vi "User_Metadata.vi"() -> ()   [LabVIEW 2020]
uses:
  ADAM Controls/Channel_names.ctl
  ADAM Controls/Calib_type_ADAM.ctl
  Anemometry/Anemometry Sub Vis/Controls/Preference_Mode.ctl
  ADAM Controls/Channel_State.ctl
  ADAM Controls/Module_type_ADAM.ctl
  ADAM Controls/Update_scan_value.ctl
  Anemometry/Anemometry Sub Vis/Globals/Preference_global.vi
  Anemometry/Anemometry Sub Vis/Globals/Constants_global.vi
  Anemometry/Anemometry Sub Vis/Globals/Meas_global.vi
  Anemometry/Anemometry Sub Vis/Globals/Trav_pos_global.vi
panel:
  out "Channel Name 13":string
  out "Channel Name 12":string
  out "Channel Name 11":string
  in  "Value 13":string
  in  "Value 12":string
  in  "Value 11":string
  in  "Menu 13":u16(ring) items=["Edit Strings", "20mm Cubes"]
  in  "Menu 12":u16(ring) items=["Edit Strings", "20mm Cubes"]
  in  "Menu 11":u16(ring) items=["Edit Strings", "20mm Cubes"]
  out "Rig Name":string="EnFlo Tunnel"
  in  "Edit Email Addresses":bool
  out "Email Addresses":string[](array[string])
  in  "Value 10":string
  in  "Value 9":string
  in  "Value 8":string
  in  "Value 7":string
  in  "Value 6":string
  in  "Menu 10":u16(ring) items=["Edit Strings", "20mm Cubes"]
  out "Channel Name 10":string
  in  "Menu 9":u16(ring) items=["Edit Strings", "None", "Ramp 29 x 390mm", "Ramp 9 x 175mm", "Rounded nose 18.2 x 55mm", "Rounded nose 9 x 150mm"]
  out "Channel Name 9":string
  in  "Menu 8":u16(ring) items=["Edit Strings", "20mm Cubes"]
  out "Channel Name 8":string
  in  "Menu 7":u16(ring) items=["Edit Strings", "0", "115", "65"]
  out "Channel Name 7":string
  in  "Menu 6":u16(ring) items=["Edit Strings", "0", "1", "16"]
  out "Channel Name 6":string
  out "Clear remaining channels":bool
  in  "Value 5":string
  in  "Menu 5":u16(ring) items=["Edit Strings", "0", "25", "6.25"]
  out "Channel Name 5":string
  in  "Value 4":string
  in  "Menu 4":u16(ring) items=["Edit Strings", "20 x 20mm", "40 x 40mm", "80 x 80mm", "None"]
  out "Channel Name 4":string
  in  "Value 3":string
  in  "Menu 3":u16(ring) items=["Edit Strings", "0", "10", "20", "Normal distribution with average = 10mm"]
  out "Channel Name 3":string
  in  "Value 2":string
  in  "Menu 2":u16(ring) items=["Edit Strings", "None", "Random blocks", "Uniform cube"]
  out "Channel Name 2":string
  in  "Modify User Channels":bool
  out "Channel No":i32
  out "First Loop":bool
  out "Index":i32
  in  "Value 1":string
  in  "Menu 1":u16(ring) items=["Edit Strings", "Aligned", "None", "Staggered"]
  out "Channel Name 1":string
  in  "stop":bool
  in  "OK":bool
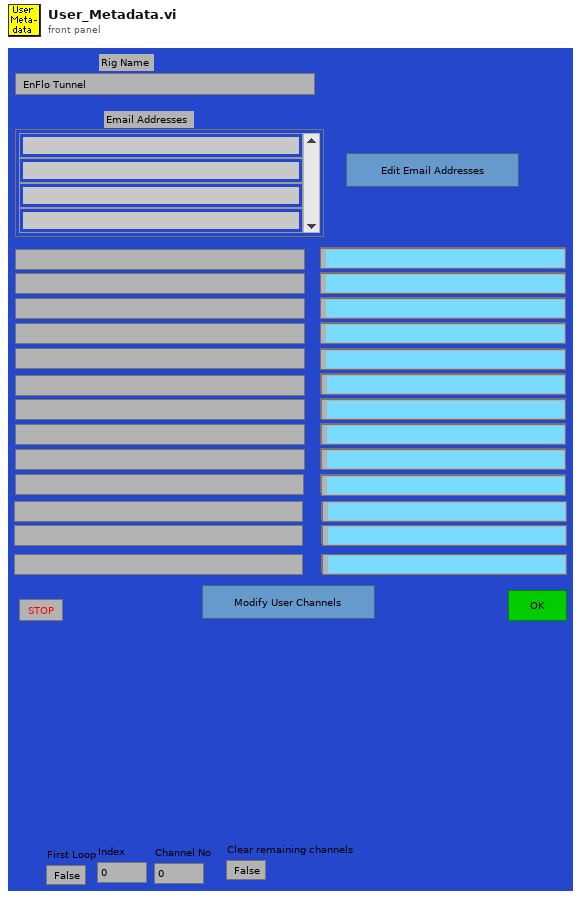
[diagram p1: front panel]
types:
  T1 = typedef "Channel_names.ctl" = enum16{"Active Only", "Active + Off", "All Channels"}
  T2 = typedef "Calib_type_ADAM.ctl" = string
  T3 = typedef "Preference_Mode.ctl" = enum16{"Load Preferences from file", "Save Preferences to file", "Load, Edit then Save"}
  T4 = typedef "Channel_State.ctl" = enum16{"On", "Off", "Always On", "Always Off"}
  T5 = typedef "Module_type_ADAM.ctl" = string
  T6 = typedef "Ch_description_ADAM.ctl" = cluster{"Ch Name":string, "Type":T5, "Function":T7, "Ch State":T4, "Calibration type":T2, "A":dbl, "B":dbl, "C":dbl, "D":dbl, "Comments":string, "Address":T8, "String":string, "Duty":u16}
  T7 = typedef "Function_ADAM.ctl" = enum16{"Analogue Input", "Digital Input", "Event counter", "Event rate", "Analogue Output", "Digital Output", "Relay Output"}
  T8 = typedef "Address.ctl" = cluster{"Main":i32, "Ch.":i32, "Sub":i32, "Port Name":string}
  T9 = typedef "Update_scan_value.ctl" = cluster{"Channel Name":string, "New Value":dbl}
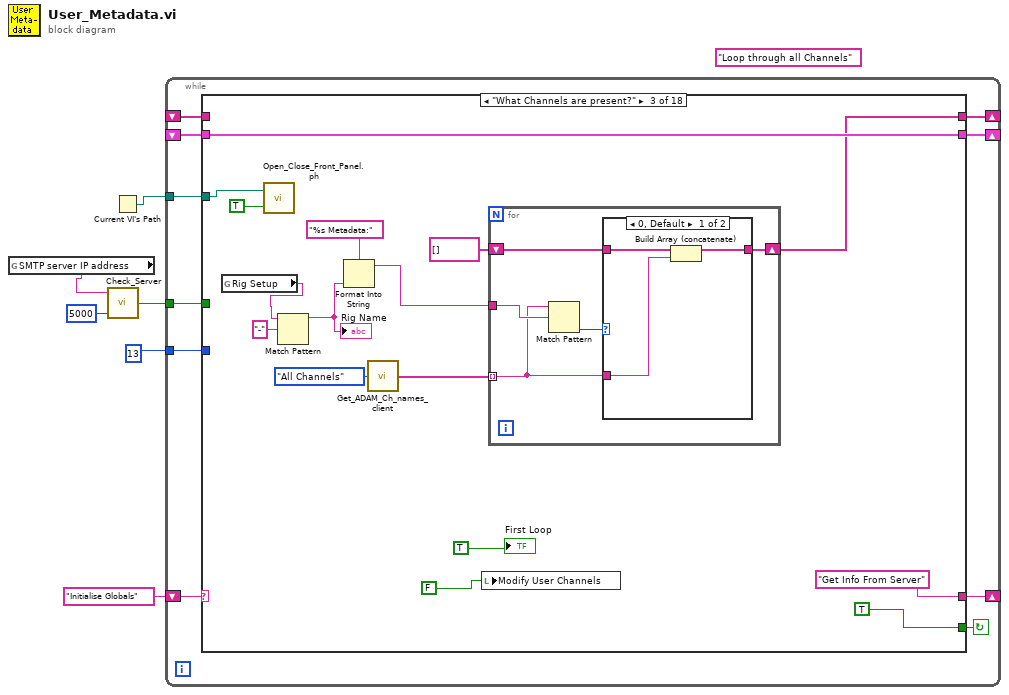
[diagram p0: block diagram]
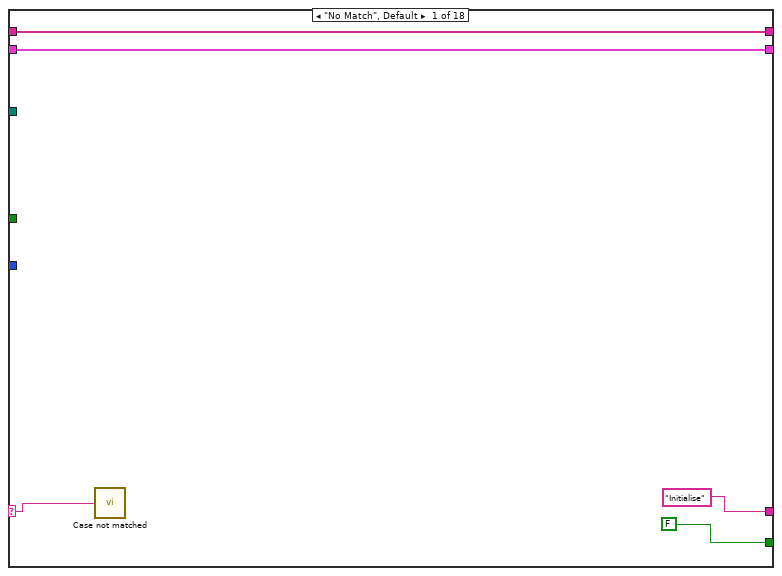
[diagram p2: hidden frame]
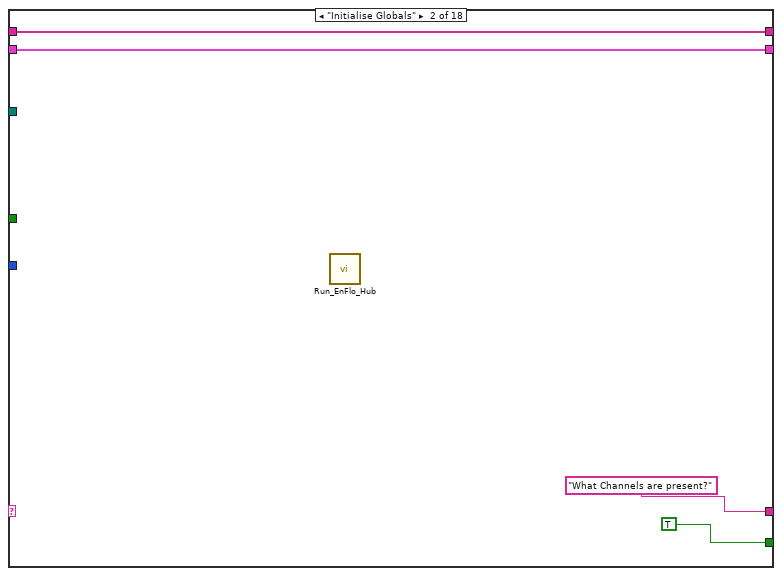
[diagram p3: hidden frame]
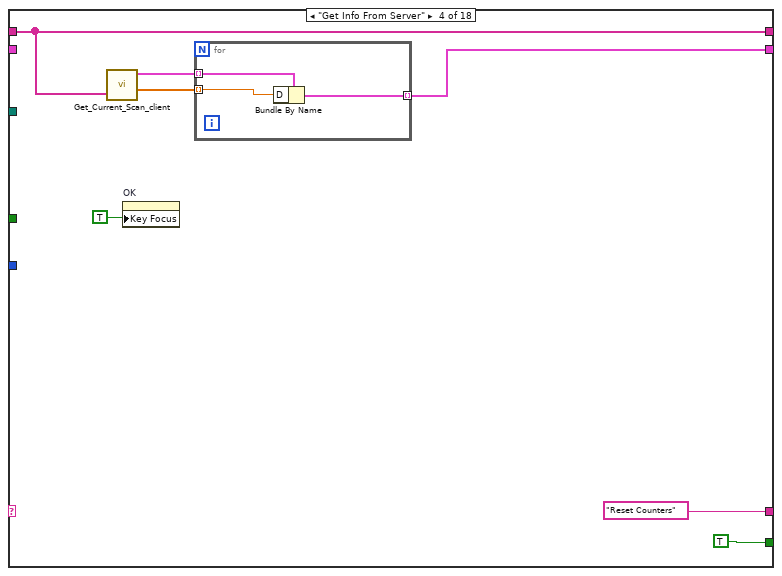
[diagram p5: hidden frame]
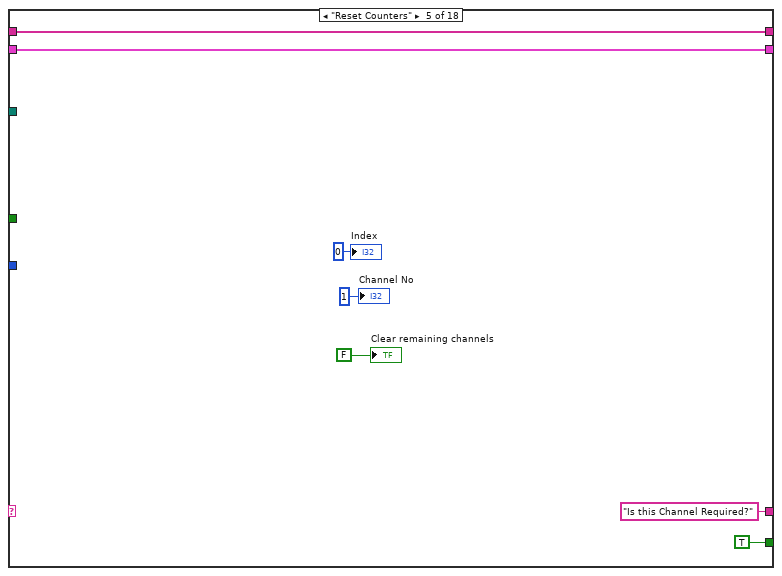
[diagram p6: hidden frame]
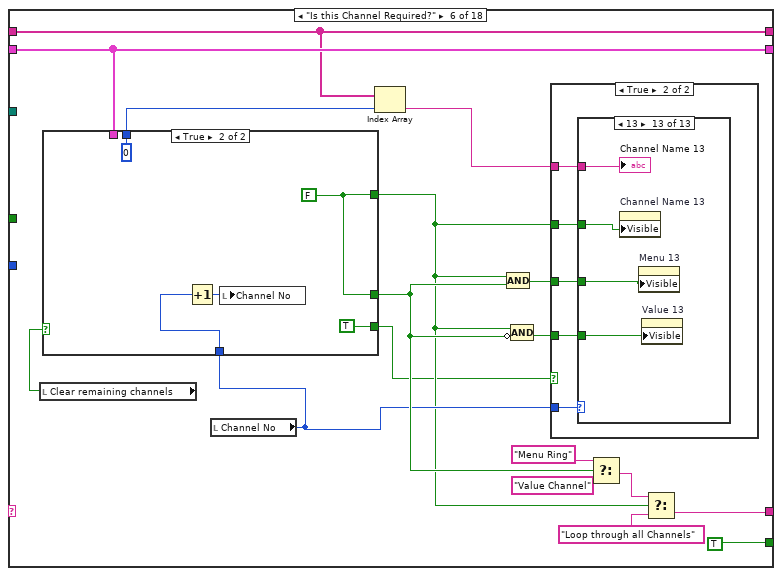
[diagram p7: hidden frame]
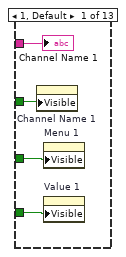
[diagram p9: hidden frame]
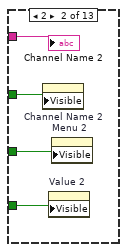
[diagram p10: hidden frame]
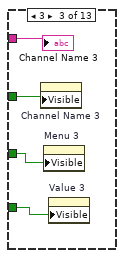
[diagram p11: hidden frame]
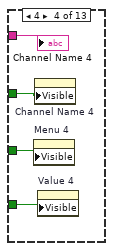
[diagram p12: hidden frame]
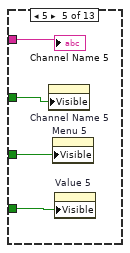
[diagram p13: hidden frame]
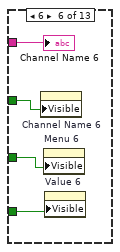
[diagram p14: hidden frame]
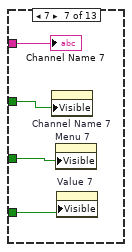
[diagram p15: hidden frame]
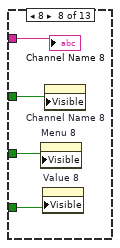
[diagram p16: hidden frame]
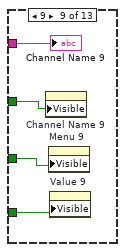
[diagram p17: hidden frame]
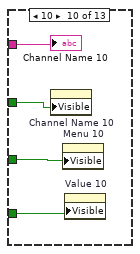
[diagram p18: hidden frame]
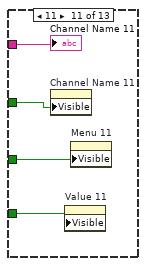
[diagram p19: hidden frame]
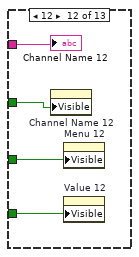
[diagram p20: hidden frame]
diagram:
  (unwired) "Loop through all Channels"
  n1 = global read "Preference_global.vi" "SMTP server IP address"() -> (w2:string)
  n2 = call "Check_Server.vi"("timeout ms (60000)"=5000, "address"=w2) -> ("OK"=w1:bool)  [unwired: 3 out]
  n3 = Current VI's Path() -> (path=w4:path)
  n4 = while {
    tunnel: 13 -> [w9]
    shift-left: _ -> [w12]
    shift-right: [w11] -> _
    shift-left: _ -> [w13]
    shift-right: [w14] -> _
    shift-left: "Initialise Globals" -> [w15]
    shift-right: [w10] -> _
    tunnel: w4 -> [w8]
    tunnel: w1 -> [w7]
    stop <- w16 continue-if-true
    n5 = case shown="\"What Channels are present?\"" w15 {
      selector: w15 -> [w17 _ _ _ _ _ _ _ _ _ _ _ _ _ _ _ _ _]
      tunnel: [FALSE TRUE TRUE TRUE TRUE ("T button?") TRUE TRUE TRUE TRUE TRUE TRUE TRUE TRUE TRUE ("T button?") TRUE ("T button?") TRUE ("T button?") TRUE ("T button?") FALSE ("T button?")] -> w16
      tunnel: ["Initialise" "What Channels are present?" "Get Info From Server" "Reset Counters" "Is this Channel Required?" w79 w173 "Increment Channel No" "Increment Channel No" "Loop through all Channels" w393 "What Channels are present?" "Reset Counters" w440 "Insert Values" "Update Server" w472 "End"] -> w10
      tunnel: [w19 w23 w39 w52 w64 w83 w165 w300 w321 w391 w404 w425 w430 w450 w457 w460 w473 w517] -> w14
      tunnel: w13 -> [w19 w23 w39 _ w64 w83 w166 w299 w322 w391 w404 w425 w431 w450 w457 w458 w473 w517]
      tunnel: w12 -> [w18 w22 _ w55 w65 w73 w185 w304 w332 w390 w409 w426 _ w443 w455 w459 w474 w518]
      tunnel: [w18 w22 w35 w55 w65 w73 w185 w304 w332 w390 w409 w426 w429 w443 w455 w459 w474 w518] -> w11
      tunnel: w9 -> [_ _ _ _ _ _ _ _ _ _ w399 _ _ _ _ _ _ _]
      tunnel: w8 -> [_ _ w30 _ _ _ _ _ _ _ _ _ _ _ _ _ _ w515]
      tunnel: w7 -> [_ _ _ _ _ _ _ _ _ _ _ _ _ _ _ _ _ _]
      frame "No Match", Default {
        n6 = call "Case not matched.vi"("Case Name not Matched"=w17) -> ()
      }
      frame "Initialise Globals" {
        n7 = call "Run_EnFlo_Hub.vi"() -> ()  [unwired: 1 in, 7 out]
      }
      frame "What Channels are present?" {
        n8 = global read "Preference_global.vi" "Rig Setup"() -> (w27:string)
        n9 = call "Open_Close_Front_Panel.ph.vi"("Front Panel Window:Open"=TRUE, "VI path"=w30) -> ()  [unwired: 2 out]
        n10 = Match Pattern(string=w27, regular expression="-") -> (before substring=w26:string)  [unwired: 4 out]
        "Rig Name" <- w26
        n11 = Format Into String(format string="%s Metadata:" ("Format String"), w26) -> (resulting string=w32:string)  [unwired: 2 in, 1 out]
        n12 = call "Get_ADAM_Ch_names_client.vi"("Channel names set"=Channel_names."All Channels") -> ("Ch names"=w37:string[])
        n13 = local write "Modify User Channels"(FALSE ("Add a New Channel")) -> ()
        n14 = for {
          tunnel: w32 -> [w46]
          tunnel: w37 -> [w44] mode=indexing
          shift-right: [w42] -> w35
          shift-left: string[] [] -> [w43]
          n15 = Match Pattern(string=w44, regular expression=w46) -> (offset past match=w45:i32)  [unwired: 4 out]
          n16 = case shown="0, Default" w45 {
            tunnel: w44 -> [w49 _]
            tunnel: w43 -> [w48 w50]
            tunnel: [w47 w50] -> w42
            frame 0, Default {
              n17 = Build Array (concatenate)(w48, w49) -> (w47:string[])
            }
            frame -1 {
            }
          }
        }
        "First Loop" <- TRUE ("First Loop")
      }
      frame "Get Info From Server" {
        n18 = call "Get_Current_Scan_client.vi"("multipleChannels"=w55) -> ("Ch Description Array"=w54:T6[], "Numerical Values"=w53:dbl[])  [unwired: 2 in, 1 out]
        n19 = property on="OK" class="Bool"("Key Focus"=TRUE) -> ()  [unwired: 2 in, 2 out]
        n20 = for {
          tunnel: w54 -> [w60] mode=indexing
          tunnel: w53 -> [w59] mode=indexing
          tunnel: [w58] -> w52 mode=indexing
          n21 = Bundle By Name(cluster=w60, "D"=w59) -> (w58:T6)
        }
      }
      frame "Reset Counters" {
        "Index" <- 0 ("Index")
        "Channel No" <- 1 ("Channel No")
        "Clear remaining channels" <- FALSE ("Clear remaining channels")
      }
      frame "Is this Channel Required?" {
        n22 = local read "Clear remaining channels"() -> (w71:bool)
        n23 = local read "Channel No"() -> (w70:i32)
        n24 = case shown="True" w71 {
          tunnel: w83 -> [w156 _]
          tunnel: [w142 w161] -> w69
          tunnel: [w152 w161] -> w78
          tunnel: [w151 0 ("Index")] -> w74
          tunnel: w70 -> [_ w158]
          tunnel: [w149 TRUE] -> w68
          frame False {
            n25 = local read "Index"() -> (w151:i32)
            n26 = Index Array(array=w156, index=w151) -> (element=w155:T6)
            n27 = Unbundle By Name(w155) -> ("Address.Port Name"=w146:string, "A"=w148:dbl, "Calibration type"=w153:T2)
            n28 = Equal?(x=w153, y=T2 "Text" ("Calibration Type")) -> (x = y?=w152:bool)
            n29 = Not Equal?(x="DELETE", y=w146) -> (x != y?=w143:bool)
            n30 = Equal?(x=w148, y=1.0 ("x")) -> (x = y?=w144:bool)
            n31 = And(x=w143, y=w144) -> (x .and. y?=w142:bool)
            n32 = Compound Arithmetic op=AND(w142, TRUE ("Input")) -> (w149:bool)
          }
          frame True {
            w161 = FALSE
            n33 = Increment(x=w158) -> (x+1=w159:i32)
            n34 = local write "Channel No"(w159) -> ()
          }
        }
        n35 = Index Array(array=w73, index=w74) -> (element=w72:string)
        n36 = Compound Arithmetic op=AND(w69, w78) -> (w81:bool)
        n37 = Compound Arithmetic op=AND(w69, invert w78) -> (w82:bool)
        n38 = case shown="True" w68 {
          tunnel: w82 -> [_ w89]
          tunnel: w81 -> [_ w88]
          tunnel: w69 -> [_ w87]
          tunnel: w72 -> [_ w86]
          tunnel: w70 -> [_ w85]
          frame False {
          }
          frame True {
            n39 = case shown="13" w85 {
              tunnel: w87 -> [w91 w95 w99 w103 w107 w112 w116 w120 w124 w128 w133 w137 w141]
              tunnel: w89 -> [w93 w97 w101 w105 w109 w110 w114 w118 w122 w126 w130 w134 w138]
              tunnel: w88 -> [w92 w96 w100 w104 w108 w111 w115 w119 w123 w129 w131 w135 w139]
              tunnel: w86 -> [w90 w94 w98 w102 w106 w113 w117 w121 w125 w127 w132 w136 w140]
              frame 1, Default {
                n40 = property on="Channel Name 1" class="Str"("Visible"=w91) -> ()  [unwired: 2 in, 2 out]
                n41 = property on="Menu 1" class="Ring (strict)"("Visible"=w92) -> ()  [unwired: 2 in, 2 out]
                n42 = property on="Value 1" class="Str"("Visible"=w93) -> ()  [unwired: 2 in, 2 out]
                "Channel Name 1" <- w90
              }
              frame 2 {
                n43 = property on="Channel Name 2" class="Str"("Visible"=w95) -> ()  [unwired: 2 in, 2 out]
                n44 = property on="Value 2" class="Str"("Visible"=w97) -> ()  [unwired: 2 in, 2 out]
                n45 = property on="Menu 2" class="Ring (strict)"("Visible"=w96) -> ()  [unwired: 2 in, 2 out]
                "Channel Name 2" <- w94
              }
              frame 3 {
                n46 = property on="Channel Name 3" class="Str"("Visible"=w99) -> ()  [unwired: 2 in, 2 out]
                n47 = property on="Menu 3" class="Ring (strict)"("Visible"=w100) -> ()  [unwired: 2 in, 2 out]
                n48 = property on="Value 3" class="Str"("Visible"=w101) -> ()  [unwired: 2 in, 2 out]
                "Channel Name 3" <- w98
              }
              frame 4 {
                n49 = property on="Menu 4" class="Ring (strict)"("Visible"=w104) -> ()  [unwired: 2 in, 2 out]
                n50 = property on="Channel Name 4" class="Str"("Visible"=w103) -> ()  [unwired: 2 in, 2 out]
                n51 = property on="Value 4" class="Str"("Visible"=w105) -> ()  [unwired: 2 in, 2 out]
                "Channel Name 4" <- w102
              }
              frame 5 {
                n52 = property on="Channel Name 5" class="Str"("Visible"=w107) -> ()  [unwired: 2 in, 2 out]
                n53 = property on="Menu 5" class="Ring (strict)"("Visible"=w108) -> ()  [unwired: 2 in, 2 out]
                n54 = property on="Value 5" class="Str"("Visible"=w109) -> ()  [unwired: 2 in, 2 out]
                "Channel Name 5" <- w106
              }
              frame 6 {
                n55 = property on="Channel Name 6" class="Str"("Visible"=w112) -> ()  [unwired: 2 in, 2 out]
                n56 = property on="Menu 6" class="Ring (strict)"("Visible"=w111) -> ()  [unwired: 2 in, 2 out]
                n57 = property on="Value 6" class="Str"("Visible"=w110) -> ()  [unwired: 2 in, 2 out]
                "Channel Name 6" <- w113
              }
              frame 7 {
                n58 = property on="Channel Name 7" class="Str"("Visible"=w116) -> ()  [unwired: 2 in, 2 out]
                n59 = property on="Menu 7" class="Ring (strict)"("Visible"=w115) -> ()  [unwired: 2 in, 2 out]
                n60 = property on="Value 7" class="Str"("Visible"=w114) -> ()  [unwired: 2 in, 2 out]
                "Channel Name 7" <- w117
              }
              frame 8 {
                n61 = property on="Menu 8" class="Ring (strict)"("Visible"=w119) -> ()  [unwired: 2 in, 2 out]
                n62 = property on="Value 8" class="Str"("Visible"=w118) -> ()  [unwired: 2 in, 2 out]
                n63 = property on="Channel Name 8" class="Str"("Visible"=w120) -> ()  [unwired: 2 in, 2 out]
                "Channel Name 8" <- w121
              }
              frame 9 {
                n64 = property on="Channel Name 9" class="Str"("Visible"=w124) -> ()  [unwired: 2 in, 2 out]
                n65 = property on="Menu 9" class="Ring (strict)"("Visible"=w123) -> ()  [unwired: 2 in, 2 out]
                n66 = property on="Value 9" class="Str"("Visible"=w122) -> ()  [unwired: 2 in, 2 out]
                "Channel Name 9" <- w125
              }
              frame 10 {
                n67 = property on="Channel Name 10" class="Str"("Visible"=w128) -> ()  [unwired: 2 in, 2 out]
                n68 = property on="Menu 10" class="Ring (strict)"("Visible"=w129) -> ()  [unwired: 2 in, 2 out]
                n69 = property on="Value 10" class="Str"("Visible"=w126) -> ()  [unwired: 2 in, 2 out]
                "Channel Name 10" <- w127
              }
              frame 11 {
                n70 = property on="Channel Name 11" class="Str"("Visible"=w133) -> ()  [unwired: 2 in, 2 out]
                n71 = property on="Value 11" class="Str"("Visible"=w130) -> ()  [unwired: 2 in, 2 out]
                n72 = property on="Menu 11" class="Ring (strict)"("Visible"=w131) -> ()  [unwired: 2 in, 2 out]
                "Channel Name 11" <- w132
              }
              frame 12 {
                n73 = property on="Channel Name 12" class="Str"("Visible"=w137) -> ()  [unwired: 2 in, 2 out]
                n74 = property on="Menu 12" class="Ring (strict)"("Visible"=w135) -> ()  [unwired: 2 in, 2 out]
                n75 = property on="Value 12" class="Str"("Visible"=w134) -> ()  [unwired: 2 in, 2 out]
                "Channel Name 12" <- w136
              }
              frame 13 {
                n76 = property on="Channel Name 13" class="Str"("Visible"=w141) -> ()  [unwired: 2 in, 2 out]
                n77 = property on="Menu 13" class="Ring (strict)"("Visible"=w139) -> ()  [unwired: 2 in, 2 out]
                n78 = property on="Value 13" class="Str"("Visible"=w138) -> ()  [unwired: 2 in, 2 out]
                "Channel Name 13" <- w140
              }
            }
          }
        }
        n79 = Select(t="Menu Ring", s=w78, f="Value Channel") -> (s? t:f=w76:string)
        n80 = Select(t=w76, s=w69, f="Loop through all Channels") -> (s? t:f=w79:string)
      }
      frame "Menu Ring" {
        n81 = local read "First Loop"() -> (w183:bool)
        n82 = local read "Index"() -> (w178:i32)
        n83 = Index Array(array=w166, index=w178) -> (element=w163:T6)
        n84 = Unbundle By Name(w163) -> ("String"=w184:string, "D"=w167:dbl)
        n85 = call "Get_array_values_fr_String.vi"("String Value"=w184) -> ("String array"=w171:string[])  [unwired: 1 out]
        n86 = To Unsigned Word Integer(number=w167) -> (unsigned 16bit integer=w182:u16)
        n87 = local read "Channel No"() -> (w177:i32)
        n88 = Build Array (concatenate)("Edit Strings", w171) -> (w172:string[])
        n89 = Increment(x=w182) -> (x+1=w180:u16)
        n90 = Array Size(array=w171) -> (size(s)=w170:i32)
        n91 = To Unsigned Word Integer(number=w170) -> (unsigned 16bit integer=w169:u16)
        n92 = case shown="13" w177 {
          tunnel: w183 -> [w193 w202 w210 w218 w226 w234 w242 w250 w258 w266 w274 w282 w290]
          tunnel: w180 -> [w192 w201 w209 w217 w225 w233 w241 w249 w257 w265 w273 w281 w289]
          tunnel: [w187 w197 w205 w213 w221 w229 w237 w245 w253 w261 w269 w277 w285] -> w179
          tunnel: w172 -> [w191 w195 w204 w212 w220 w227 w236 w244 w252 w260 w268 w276 w284]
          tunnel: w169 -> [w188 w198 w206 w214 w222 w230 w238 w246 w254 w262 w270 w278 w286]
          frame 1, Default {
            n93 = property on="Menu 1" class="Ring (strict)"("Strings []"=w191) -> ()  [unwired: 2 in, 2 out]
            n94 = Select(t=w192, s=w193, f="Menu 1") -> (s? t:f=w189:u16)
            n95 = Less?(x=w189, y=w188) -> (x < y?=w190:bool)
            n96 = Select(t=w189, s=w190, f=w188) -> (s? t:f=w187:u16)
            n97 = local write "Menu 1"(w187) -> ()
          }
          frame 2 {
            n98 = property on="Menu 2" class="Ring (strict)"("Strings []"=w195) -> ()  [unwired: 2 in, 2 out]
            n99 = Select(t=w201, s=w202, f="Menu 2") -> (s? t:f=w199:u16)
            n100 = Less?(x=w199, y=w198) -> (x < y?=w200:bool)
            n101 = Select(t=w199, s=w200, f=w198) -> (s? t:f=w197:u16)
            n102 = local write "Menu 2"(w197) -> ()
          }
          frame 3 {
            n103 = property on="Menu 3" class="Ring (strict)"("Strings []"=w204) -> ()  [unwired: 2 in, 2 out]
            n104 = Select(t=w209, s=w210, f="Menu 3") -> (s? t:f=w207:u16)
            n105 = Less?(x=w207, y=w206) -> (x < y?=w208:bool)
            n106 = Select(t=w207, s=w208, f=w206) -> (s? t:f=w205:u16)
            n107 = local write "Menu 3"(w205) -> ()
          }
          frame 4 {
            n108 = property on="Menu 4" class="Ring (strict)"("Strings []"=w212) -> ()  [unwired: 2 in, 2 out]
            n109 = Select(t=w217, s=w218, f="Menu 4") -> (s? t:f=w215:u16)
            n110 = Less?(x=w215, y=w214) -> (x < y?=w216:bool)
            n111 = Select(t=w215, s=w216, f=w214) -> (s? t:f=w213:u16)
            n112 = local write "Menu 4"(w213) -> ()
          }
          frame 5 {
            n113 = property on="Menu 5" class="Ring (strict)"("Strings []"=w220) -> ()  [unwired: 2 in, 2 out]
            n114 = Select(t=w225, s=w226, f="Menu 5") -> (s? t:f=w223:u16)
            n115 = Less?(x=w223, y=w222) -> (x < y?=w224:bool)
            n116 = Select(t=w223, s=w224, f=w222) -> (s? t:f=w221:u16)
            n117 = local write "Menu 5"(w221) -> ()
          }
          frame 6 {
            n118 = property on="Menu 6" class="Ring (strict)"("Strings []"=w227) -> ()  [unwired: 2 in, 2 out]
            n119 = Select(t=w233, s=w234, f="Menu 6") -> (s? t:f=w231:u16)
            n120 = Less?(x=w231, y=w230) -> (x < y?=w232:bool)
            n121 = Select(t=w231, s=w232, f=w230) -> (s? t:f=w229:u16)
            n122 = local write "Menu 6"(w229) -> ()
          }
          frame 7 {
            n123 = property on="Menu 7" class="Ring (strict)"("Strings []"=w236) -> ()  [unwired: 2 in, 2 out]
            n124 = Select(t=w241, s=w242, f="Menu 7") -> (s? t:f=w239:u16)
            n125 = Less?(x=w239, y=w238) -> (x < y?=w240:bool)
            n126 = Select(t=w239, s=w240, f=w238) -> (s? t:f=w237:u16)
            n127 = local write "Menu 7"(w237) -> ()
          }
          frame 8 {
            n128 = property on="Menu 8" class="Ring (strict)"("Strings []"=w244) -> ()  [unwired: 2 in, 2 out]
            n129 = Select(t=w249, s=w250, f="Menu 8") -> (s? t:f=w247:u16)
            n130 = Less?(x=w247, y=w246) -> (x < y?=w248:bool)
            n131 = Select(t=w247, s=w248, f=w246) -> (s? t:f=w245:u16)
            n132 = local write "Menu 8"(w245) -> ()
          }
          frame 9 {
            n133 = property on="Menu 9" class="Ring (strict)"("Strings []"=w252) -> ()  [unwired: 2 in, 2 out]
            n134 = Select(t=w257, s=w258, f="Menu 9") -> (s? t:f=w255:u16)
            n135 = Less?(x=w255, y=w254) -> (x < y?=w256:bool)
            n136 = Select(t=w255, s=w256, f=w254) -> (s? t:f=w253:u16)
            n137 = local write "Menu 9"(w253) -> ()
          }
          frame 10 {
            n138 = property on="Menu 10" class="Ring (strict)"("Strings []"=w260) -> ()  [unwired: 2 in, 2 out]
            n139 = Select(t=w265, s=w266, f="Menu 10") -> (s? t:f=w263:u16)
            n140 = Less?(x=w263, y=w262) -> (x < y?=w264:bool)
            n141 = Select(t=w263, s=w264, f=w262) -> (s? t:f=w261:u16)
            n142 = local write "Menu 10"(w261) -> ()
          }
          frame 11 {
            n143 = property on="Menu 11" class="Ring (strict)"("Strings []"=w268) -> ()  [unwired: 2 in, 2 out]
            n144 = Select(t=w273, s=w274, f="Menu 11") -> (s? t:f=w271:u16)
            n145 = Less?(x=w271, y=w270) -> (x < y?=w272:bool)
            n146 = Select(t=w271, s=w272, f=w270) -> (s? t:f=w269:u16)
            n147 = local write "Menu 11"(w269) -> ()
          }
          frame 12 {
            n148 = property on="Menu 12" class="Ring (strict)"("Strings []"=w276) -> ()  [unwired: 2 in, 2 out]
            n149 = Select(t=w281, s=w282, f="Menu 12") -> (s? t:f=w279:u16)
            n150 = Less?(x=w279, y=w278) -> (x < y?=w280:bool)
            n151 = Select(t=w279, s=w280, f=w278) -> (s? t:f=w277:u16)
            n152 = local write "Menu 12"(w277) -> ()
          }
          frame 13 {
            n153 = property on="Menu 13" class="Ring (strict)"("Strings []"=w284) -> ()  [unwired: 2 in, 2 out]
            n154 = Select(t=w289, s=w290, f="Menu 13") -> (s? t:f=w287:u16)
            n155 = Less?(x=w287, y=w286) -> (x < y?=w288:bool)
            n156 = Select(t=w287, s=w288, f=w286) -> (s? t:f=w285:u16)
            n157 = local write "Menu 13"(w285) -> ()
          }
        }
        n158 = Equal To 0?(x=w179) -> (x = 0?=w176:bool)
        n159 = Select(t="Edit Menu Strings", s=w176, f="Increment Channel No") -> (s? t:f=w173:string)
        n160 = Decrement(x=w179) -> (x-1=w168:u16)
        n161 = To Double Precision Float(number=w168) -> (double precision float=w164:dbl)
        n162 = Bundle By Name(cluster=w163, "D"=w164) -> (w162:T6)
        n163 = Replace Array Subset(array=w166, new element=w162, index=w178) -> (w165:T6[])
      }
      frame "Edit Menu Strings" {
        n164 = local read "Index"() -> (w294:i32)
        n165 = Index Array(array=w299, index=w294) -> (element=w303:T6)
        n166 = Unbundle By Name(w303) -> ("String"=w305:string, "Ch Name"=w293:string)
        n167 = call "Get_array_values_fr_String.vi"("String Value"=w305) -> ("String array"=w298:string[])  [unwired: 1 out]
        n168 = call "Edit_String_Options_list.vi"("Channel Name"=w293, "String array"=w298) -> ("New Selection Index"=w291:i32, "String array Out"=w297:string[])
        n169 = call "Put_Array_into_String.vi"("String array"=w297) -> ("String Value"=w302:string)
        n170 = local read "Channel No"() -> (w296:i32)
        n171 = Increment(x=w291) -> (x+1=w295:i32)
        n172 = Bundle By Name(cluster=w303, "String"=w302, "D"=w291) -> (w301:T6)
        n173 = To Unsigned Word Integer(number=w295) -> (unsigned 16bit integer=w292:u16)
        n174 = case shown="1, Default" w296 {
          tunnel: w292 -> [w308 w309 w310 w311 w312 w313 w314 w315 w316 w317 w318 w319 w320]
          frame 1, Default {
            n175 = local write "Menu 1"(w308) -> ()
          }
          frame 2 {
            n176 = local write "Menu 2"(w309) -> ()
          }
          frame 3 {
            n177 = local write "Menu 3"(w310) -> ()
          }
          frame 4 {
            n178 = local write "Menu 4"(w311) -> ()
          }
          frame 5 {
            n179 = local write "Menu 5"(w312) -> ()
          }
          frame 6 {
            n180 = local write "Menu 6"(w313) -> ()
          }
          frame 7 {
            n181 = local write "Menu 7"(w314) -> ()
          }
          frame 8 {
            n182 = local write "Menu 8"(w315) -> ()
          }
          frame 9 {
            n183 = local write "Menu 9"(w316) -> ()
          }
          frame 10 {
            n184 = local write "Menu 10"(w317) -> ()
          }
          frame 11 {
            n185 = local write "Menu 11"(w318) -> ()
          }
          frame 12 {
            n186 = local write "Menu 12"(w319) -> ()
          }
          frame 13 {
            n187 = local write "Menu 13"(w320) -> ()
          }
        }
        n188 = Replace Array Subset(array=w299, new element=w301, index=w294) -> (w300:T6[])
      }
      frame "Value Channel" {
        n189 = local read "Index"() -> (w331:i32)
        n190 = local read "First Loop"() -> (w329:bool)
        n191 = Index Array(array=w322, index=w331) -> (element=w323:T6)
        n192 = local read "Channel No"() -> (w330:i32)
        n193 = Unbundle By Name(w323) -> ("D"=w325:dbl)
        n194 = call "Number_2_string.vi"("number"=w325) -> ("String"=w328:string)  [unwired: 1 in]
        n195 = case shown="1, Default" w330 {
          tunnel: w329 -> [w338 w342 w346 w350 w354 w358 w362 w366 w370 w374 w378 w382 w386]
          tunnel: w328 -> [w337 w341 w345 w349 w353 w357 w361 w365 w369 w373 w377 w381 w385]
          tunnel: [w335 w340 w344 w348 w352 w356 w360 w364 w368 w372 w376 w380 w384] -> w327
          frame 1, Default {
            n196 = Select(t=w337, s=w338, f="Value 1") -> (s? t:f=w335:string)
            n197 = local write "Value 1"(w335) -> ()
          }
          frame 2 {
            n198 = Select(t=w341, s=w342, f="Value 2") -> (s? t:f=w340:string)
            n199 = local write "Value 2"(w340) -> ()
          }
          frame 3 {
            n200 = Select(t=w345, s=w346, f="Value 3") -> (s? t:f=w344:string)
            n201 = local write "Value 3"(w344) -> ()
          }
          frame 4 {
            n202 = Select(t=w349, s=w350, f="Value 4") -> (s? t:f=w348:string)
            n203 = local write "Value 4"(w348) -> ()
          }
          frame 5 {
            n204 = Select(t=w353, s=w354, f="Value 5") -> (s? t:f=w352:string)
            n205 = local write "Value 5"(w352) -> ()
          }
          frame 6 {
            n206 = Select(t=w357, s=w358, f="Value 6") -> (s? t:f=w356:string)
            n207 = local write "Value 6"(w356) -> ()
          }
          frame 7 {
            n208 = Select(t=w361, s=w362, f="Value 7") -> (s? t:f=w360:string)
            n209 = local write "Value 7"(w360) -> ()
          }
          frame 8 {
            n210 = Select(t=w365, s=w366, f="Value 8") -> (s? t:f=w364:string)
            n211 = local write "Value 8"(w364) -> ()
          }
          frame 9 {
            n212 = Select(t=w369, s=w370, f="Value 9") -> (s? t:f=w368:string)
            n213 = local write "Value 9"(w368) -> ()
          }
          frame 10 {
            n214 = Select(t=w373, s=w374, f="Value 10") -> (s? t:f=w372:string)
            n215 = local write "Value 10"(w372) -> ()
          }
          frame 11 {
            n216 = Select(t=w377, s=w378, f="Value 11") -> (s? t:f=w376:string)
            n217 = local write "Value 11"(w376) -> ()
          }
          frame 12 {
            n218 = Select(t=w381, s=w382, f="Value 12") -> (s? t:f=w380:string)
            n219 = local write "Value 12"(w380) -> ()
          }
          frame 13 {
            n220 = Select(t=w385, s=w386, f="Value 13") -> (s? t:f=w384:string)
            n221 = local write "Value 13"(w384) -> ()
          }
        }
        n222 = Fract/Exp String To Number(string=w327) -> (number=w326:dbl)  [unwired: 4 out]
        n223 = Bundle By Name(cluster=w323, "D"=w326) -> (w324:T6)
        n224 = Replace Array Subset(array=w322, new element=w324, index=w331) -> (w321:T6[])
      }
      frame "Increment Channel No" {
        n225 = local read "Channel No"() -> (w389:i32)
        n226 = Increment(x=w389) -> (x+1=w388:i32)
        n227 = local write "Channel No"(w388) -> ()
      }
      frame "Loop through all Channels" {
        n228 = local read "Index"() -> (w408:i32)
        n229 = Array Size(array=w404) -> (size(s)=w403:i32)
        n230 = local read "Channel No"() -> (w394:i32)
        n231 = Increment(x=w408) -> (x+1=w407:i32)
        n232 = Less?(x=w407, y=w403) -> (x < y?=w397:bool)
        n233 = local write "Index"(w407) -> ()
        n234 = Less Or Equal?(x=w394, y=w399) -> (x <= y?=w396:bool)
        n235 = Or(x=w397, y=w396) -> (x .or. y?=w398:bool)
        n236 = Compound Arithmetic op=AND(invert w397, w396) -> (w395:bool)
        n237 = case shown="False" w395 {
          frame False {
          }
          frame True {
            n238 = local write "Clear remaining channels"(TRUE ("Clear remaining channels")) -> ()
          }
        }
        n239 = Select(t="Is this Channel Required?", s=w398, f="Is User Ready Yet?") -> (s? t:f=w400:string)
        n240 = Select(t="Edit User Channels", s="Modify User Channels", f=w400) -> (s? t:f=w393:string)
      }
      frame "Edit Preference Panel" {
        n241 = global read "Constants_global.vi" "EnFlo SW Folder"() -> (w413:path)
        n242 = Build Path(base path=w413, name or relative path=path "Anemometry/Utilities/Preference_Panel.vi") -> (appended path=w416:path)
        n243 = Open VI Reference(type specifier VI Refnum (for type only)=refnum<vi> refnum, vi path=w416) -> (vi reference=w423:refnum<vi>, error out=w422:errorcluster)  [unwired: 1 in, 3 out]
        n244 = property class="VI Interface Type 2"(reference=w423, error in=w422, "Front Panel Window:Open"=TRUE) -> (reference out=w420:refnum<vi>, error out=w419:errorcluster)
        n245 = call-by-ref "?"(reference=w420, error in=w419, "Mode"=Preference_Mode."Load, Edit then Save") -> (reference out=w418:refnum<vi>, error out=w417:errorcluster)
        n246 = Close Reference(reference=w418, error in (no error)=w417) -> ()  [unwired: 1 out]
      }
      frame "Edit User Channels" {
        n247 = call "Modify_Metadata_Channels.vi"("Ch Description Array"=w431) -> ("Ch Description Array Out"=w430:T6[])  [unwired: 4 out]
        n248 = local write "First Loop"(TRUE ("First Loop")) -> ()
        n249 = for {
          tunnel: w430 -> [w436] mode=indexing
          tunnel: [w435] -> w429 mode=indexing
          n250 = Unbundle By Name(w436) -> ("Ch Name"=w435:string)
        }
        n251 = local write "Modify User Channels"(FALSE ("Add a New Channel")) -> ()
      }
      frame "Is User Ready Yet?" {
        w442 = FALSE ("First Loop")
        n252 = Or(x="stop", y="OK") -> (x .or. y?=w446:bool)
        n253 = case shown="True" "Edit Email Addresses" {
          frame False {
            n254 = global read "Meas_global.vi" "People to Email"() -> (→"Email Addresses":string[])
          }
          frame True {
            w452 = FALSE  # OK
            n255 = call "Get_users_email_addresses.vi"("OK"=w452) -> ()  [unwired: 5 out]
            n256 = local write "Edit Email Addresses"(FALSE ("Edit Email Addresses")) -> ()
          }
        }
        n257 = Current VI's Path() -> (path=w448:path)
        n258 = call "Close_Panel_and_Abort.vi"("Vi path"=w448, "stop"="stop") -> ()  [unwired: 1 out]
        n259 = Select(t="Valid User Name?", s=w446, f="Reset Counters") -> (s? t:f=w438:string)
        n260 = Select(t="Insert Values", s="stop", f=w438) -> (s? t:f=w440:string)
        n261 = local write "Clear remaining channels"(w442) -> ()
        n262 = local write "First Loop"(w442) -> ()
      }
      frame "Valid User Name?" {
      }
      frame "Insert Values" {
        n263 = for {
          tunnel: w458 -> [w469] mode=indexing
          tunnel: [w463] -> w460 mode=indexing
          n264 = Unbundle By Name(w469) -> ("A"=w471:dbl)
          n265 = Equal?(x=1.0, y=w471) -> (x = y?=w467:bool)
          n266 = Select(t=Channel_State."On" ("Channel State"), s=w467, f=Channel_State."Off" ("Channel State")) -> (s? t:f=w464:T4)
          n267 = Bundle By Name(cluster=w469, "Type"=T5 "Hold Value" ("Module Type"), "Ch State"=w464) -> (w463:T6)
        }
      }
      frame "Update Server" {
        n268 = stacked-sequence {
          seq-local: [w478 _] -> [_ _]
          seq-local: [w476 _] -> [_ _]
          tunnel: w473 -> [w484 _]
          tunnel: [_ "Close Panel"] -> w472
          frame #0 {
            w482 = T9 {"Channel Name"="", "New Value"=0.0} ("Update Scan Value Cluster")
            n269 = call "Update_Ch_Discription_client.vi"("Channels to update In"=w484) -> ()  [unwired: 1 out]
            n270 = Initialize Array(w482, 0 ("dimension size")) -> (w483:T9[])
            n271 = for {
              tunnel: w482 -> [w498]
              tunnel: w484 -> [w497] mode=indexing
              shift-right: [w490] -> w480
              shift-left: w483 -> [w491]
              shift-right: [w487] -> w478
              shift-left: i32[] [] -> [w488]
              shift-right: [w485] -> w476
              shift-left: dbl[] [] -> [w486]
              i -> [w489]
              n272 = Unbundle By Name(w497) -> ("Address.Port Name"=w494:string, "Ch Name"=w495:string, "D"=w496:dbl)
              n273 = Not Equal?(x="DELETE", y=w494) -> (x != y?=w492:bool)
              n274 = case shown="True" w492 {
                tunnel: w498 -> [_ w512]
                tunnel: w496 -> [_ w504]
                tunnel: w495 -> [_ w511]
                tunnel: w491 -> [w501 w510]
                tunnel: [w501 w509] -> w490
                tunnel: w489 -> [_ w507]
                tunnel: w488 -> [w500 w506]
                tunnel: [w500 w505] -> w487
                tunnel: w486 -> [w499 w503]
                tunnel: [w499 w502] -> w485
                frame False {
                }
                frame True {
                  n275 = Bundle By Name(cluster=w512, "Channel Name"=w511, "New Value"=w504) -> (w508:T9)
                  n276 = Build Array (concatenate)(w510, w508) -> (w509:T9[])
                  n277 = Build Array (concatenate)(w506, w507) -> (w505:i32[])
                  n278 = Build Array (concatenate)(w503, w504) -> (w502:dbl[])
                }
              }
            }
            n279 = call "Update_Current_Value_client.vi"("Update array in"=w480) -> ()  [unwired: 1 in]
          }
          frame #1 {
          }
        }
      }
      frame "Close Panel" {
        n280 = call "Open_Close_Front_Panel.ph.vi"("Front Panel Window:Open"=FALSE, "VI path"=w515) -> ()  [unwired: 2 out]
        n281 = global write "Trav_pos_global.vi" "Show User Metadata on Launch?"(FALSE) -> ()
      }
    }
  }
